vi "HTTP-SetVersion.vi"(8 "error in (no error)":errorcluster, 11 "ByteGSWebAPI-V0 in":refnum<class "ByteGSWebAPI-V0.lvclass">) -> (0 "error out":errorcluster, 3 "ByteGSWebAPI-V0 out":refnum<class "ByteGSWebAPI-V0.lvclass">)   [LabVIEW 2019, in "ByteGSWebAPI.lvlib" / "ByteGSWebAPI-V0.lvclass"]
doc: "Setta la versione della richiesta nell'header HTTP"
uses:
  ByteGSWebAPI-V0.lvclass
  ByteGSWebAPI-V0.lvclass/ByteGSWebAPI-V0.ctl
  <vilib>/httpClient/LabVIEWHTTPClient.lvlib
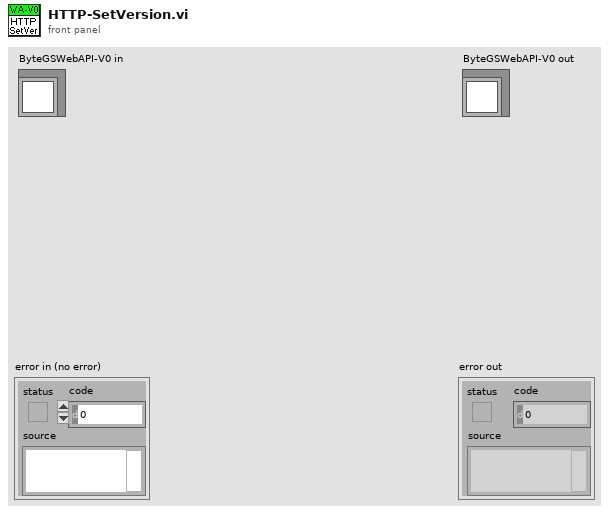
[diagram p1: front panel]
types:
  T1 = typedef "LabVIEWHTTPClient.lvlib/ClientHandle.ctl" = refnum<k1>
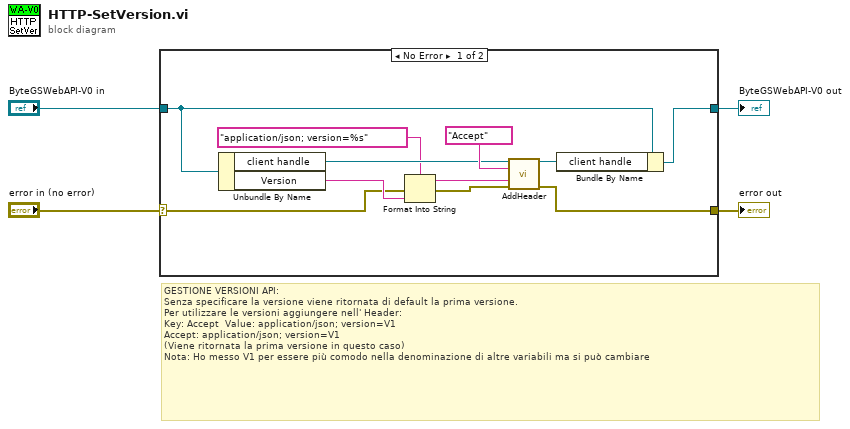
[diagram p0: block diagram]
diagram:
  # "GESTIONE VERSIONI API:\nSenza specificare la versione viene ritornata di default la prima versione.\nPer utilizzare le versioni aggiungere nell' Header:\nKey: Accept\t\tValue: application/json; version=V1\nAccept: application/json; version=V1\n(Viene ritornata la prima versione in questo caso)\nNota: Ho messo V1 per essere più comodo nella denominazione di altre variabili ma si può cambiare"
  n1 = case shown="No Error" "error in (no error)" {
    selector: "error in (no error)" -> [w5 w17]
    tunnel: [w10 w17] -> w3
    tunnel: [w12 w16] -> w1
    tunnel: "ByteGSWebAPI-V0 in" -> [w14 w16]
    frame No Error {
      n2 = Unbundle By Name(w14) -> ("client handle"=w13:T1, "Version"=w8:string)
      n3 = Format Into String(format string="application/json; version=%s" ("Version"), error in=w5, w8) -> (resulting string=w7:string, error out=w6:errorcluster)  [unwired: 1 in]
      n4 = call <vilib>:"AddHeader.vi"("client handle"=w13, "header"="Accept", "value"=w7, "error in (no error)"=w6) -> ("client handle out"=w11:T1, "error out"=w10:errorcluster)  [unwired: 10 in]
      n5 = Bundle By Name(cluster=w14, "client handle"=w11) -> (w12:refnum<class "ByteGSWebAPI-V0.lvclass">)
    }
    frame Error {
    }
  }
  "error out" <- w3
  "ByteGSWebAPI-V0 out" <- w1
